vi "PPAS_Command_Execute.vi"(8 "error in (no error)":errorcluster) -> (0 "error out":errorcluster)   [LabVIEW 2019]
uses:
  <vilib>/Rock Robotics/WPI/ThirdParty/JAS_Junk/TrajLib/VI/BoolCmd_Recv_Internal.vi
  <vilib>/Rock Robotics/WPI/ThirdParty/JAS_Junk/TrajLib/VI/BoolCmd_ObtainQueue.vi
  <vilib>/Rock Robotics/Network Tables/NT Write Boolean.vi
  PPAS_Command_Globals.vi
  <vilib>/Rock Robotics/WPI/ThirdParty/JAS_Junk/TrajLib/Trajectory_Library.lvlib
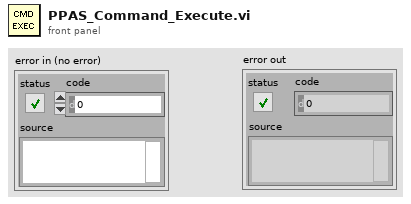
[diagram p1: front panel]
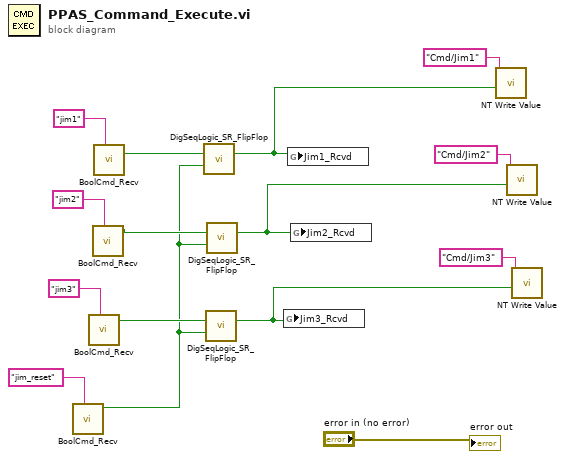
[diagram p0: block diagram]
diagram:
  n1 = call <vilib>:"BoolCmd_Recv.vi"("Command Name"="jim_reset") -> ("New Request"=w5:bool)  [unwired: 9 in, 1 out]
  n2 = call <vilib>:"BoolCmd_Recv.vi"("Command Name"="jim3") -> ("New Request"=w10:bool)  [unwired: 9 in, 1 out]
  n3 = call <vilib>:"BoolCmd_Recv.vi"("Command Name"="jim2") -> ("New Request"=w12:bool)  [unwired: 9 in, 1 out]
  n4 = call <vilib>:"BoolCmd_Recv.vi"("Command Name"="jim1") -> ("New Request"=w11:bool)  [unwired: 9 in, 1 out]
  n5 = call <vilib>:"DigSeqLogic_SR_FlipFlop.vi"("Set"=w11, "Reset"=w5) -> ("Output"=w3:bool)  [unwired: 12 in, 1 out]
  n6 = call <vilib>:"DigSeqLogic_SR_FlipFlop.vi"("Set"=w10, "Reset"=w5) -> ("Output"=w1:bool)  [unwired: 12 in, 1 out]
  n7 = call <vilib>:"DigSeqLogic_SR_FlipFlop.vi"("Set"=w12, "Reset"=w5) -> ("Output"=w2:bool)  [unwired: 12 in, 1 out]
  n8 = global write "PPAS_Command_Globals.vi" "Jim3_Rcvd"(w1) -> ()
  n9 = global write "PPAS_Command_Globals.vi" "Jim1_Rcvd"(w3) -> ()
  n10 = global write "PPAS_Command_Globals.vi" "Jim2_Rcvd"(w2) -> ()
  n11 = call-poly <vilib>:"NT Write Value.vi"("value"=w3, "name"="Cmd/Jim1") -> ()  [unwired: 9 in, 1 out]
  n12 = call-poly <vilib>:"NT Write Value.vi"("value"=w2, "name"="Cmd/Jim2") -> ()  [unwired: 9 in, 1 out]
  n13 = call-poly <vilib>:"NT Write Value.vi"("value"=w1, "name"="Cmd/Jim3") -> ()  [unwired: 9 in, 1 out]
  "error out" <- "error in (no error)"
